vi "HRM-process-manual_heartrate.vi"(9 "Bottom":dbl, 10 "Top":dbl, 11 "data in":waveform(dbl)) -> (3 "Frequency [Hz]":dbl)   [LabVIEW 2020]
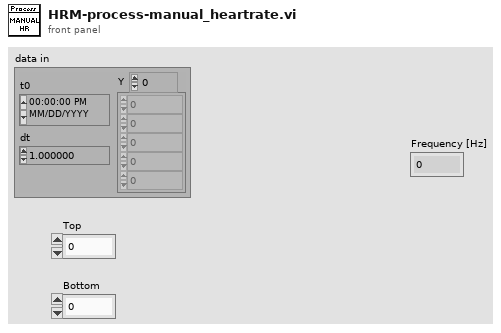
[diagram p1: front panel]
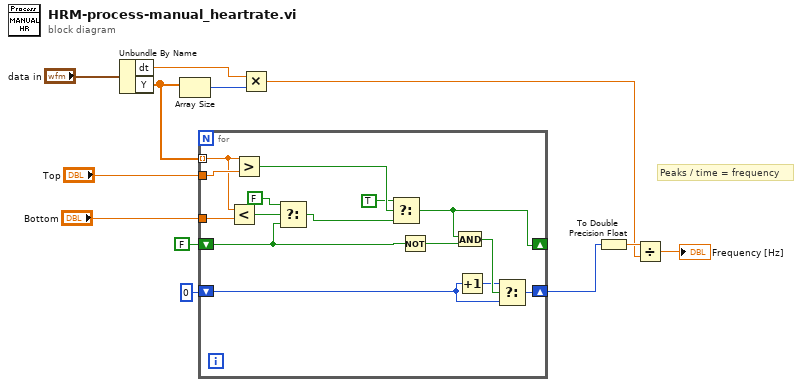
[diagram p0: block diagram]
diagram:
  # "Peaks / time = frequency"
  n1 = Unbundle By Name("data in") -> ("dt"=w6:dbl, "Y"=w7:dbl[])
  n2 = Array Size(array=w7) -> (size(s)=w5:i32)
  n3 = for {
    tunnel: "Top" -> [w27]
    tunnel: w7 -> [w23] mode=indexing
    tunnel: "Bottom" -> [w24]
    shift-right: [w19] -> _
    shift-left: FALSE ("s") -> [w18]
    shift-right: [w13] -> w2
    shift-left: 0 -> [w14]
    n4 = Less?(x=w23, y=w24) -> (x < y?=w22:bool)
    n5 = Greater?(x=w23, y=w27) -> (0:w26:bool)
    n6 = Select(t=FALSE, s=w22, f=w18) -> (s? t:f=w20:bool)
    n7 = Select(t=TRUE ("s"), s=w26, f=w20) -> (s? t:f=w19:bool)
    n8 = Not(x=w18) -> (.not. x?=w17:bool)
    n9 = And(x=w19, y=w17) -> (x .and. y?=w16:bool)
    n10 = Increment(x=w14) -> (x+1=w15:i32)
    n11 = Select(t=w15, s=w16, f=w14) -> (s? t:f=w13:i32)
  }
  n12 = Multiply(x=w6, y=w5) -> (x*y=w1:dbl)
  n13 = To Double Precision Float(number=w2) -> (double precision float=w3:dbl)
  n14 = Divide(x=w3, y=w1) -> (x/y=→"Frequency [Hz]":dbl)
